vi "TouchPanel.MainTest.vi"(11 "VI ref":refnum<vi>) -> (2 "Label.Text":string, 3 "control used?":bool)   [LabVIEW 2013]
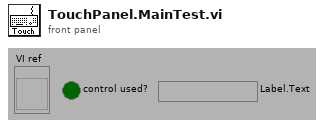
[diagram p1: front panel]
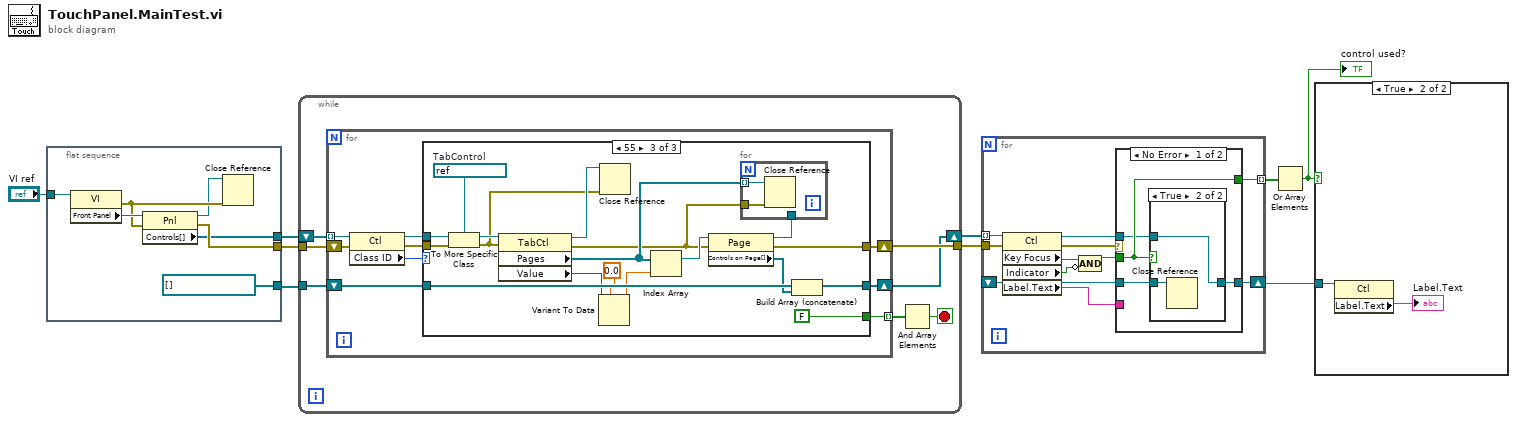
[diagram p0: block diagram]
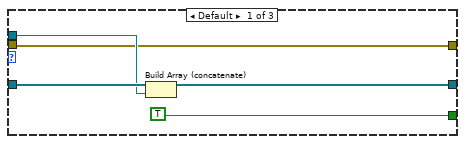
[diagram p2: hidden frame]
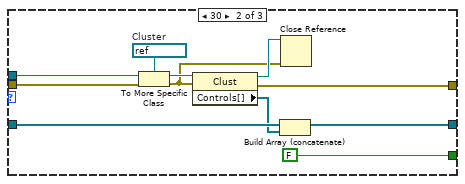
[diagram p3: hidden frame]
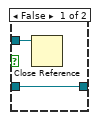
[diagram p5: hidden frame]
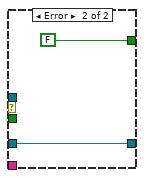
[diagram p6: hidden frame]
diagram:
  n1 = flat-sequence {
    tunnel: [w13] -> w7
    tunnel: [refnum<vi>[] []] -> w5
    tunnel: [w11] -> w4
    tunnel: "VI ref" -> [w10]
    frame #0 {
      n2 = property class="VI"(reference=w10) -> (error out=w15:errorcluster, "Front Panel"=w16:refnum<vi>)  [unwired: 1 in, 1 out]
      n3 = property class="Pnl"(reference=w16, error in=w15) -> (reference out=w14:refnum<vi>, error out=w13:errorcluster, "Controls[]"=w11:refnum<vi>[])
      n4 = Close Reference(reference=w14, error in (no error)=w15) -> ()  [unwired: 1 out]
    }
  }
  n5 = while {
    tunnel: w7 -> [w23]
    tunnel: [w22] -> w6
    tunnel: w5 -> [w21]
    shift-right: [w19] -> w3
    shift-left: w4 -> [w20]
    stop <- w17 stop-if-true
    n6 = for {
      tunnel: w20 -> [w32] mode=indexing
      shift-right: [w26] -> w22
      shift-left: w23 -> [w31]
      shift-right: [w27] -> w19
      shift-left: w21 -> [w28]
      tunnel: [w24] -> w18 mode=indexing
      n7 = property class="Ctl"(reference=w32, error in=w31) -> (reference out=w30:refnum<vi>, error out=w29:errorcluster, "Class ID"=w25:u32)
      n8 = case shown="55" w25 {
        tunnel: w30 -> [w36 w46 w65]
        tunnel: w29 -> [w34 w45 w64]
        tunnel: w28 -> [w37 w42 w60]
        tunnel: [w35 w40 w59] -> w27
        tunnel: [w34 w39 w58] -> w26
        tunnel: [TRUE FALSE FALSE] -> w24
        frame Default {
          n9 = Build Array (concatenate)(w37, w36) -> (w35:refnum<vi>[])
        }
        frame 30 {
          w47 = refnum<vi> refnum  # Cluster
          n10 = To More Specific Class(target class=w47, reference=w46, error in=w45) -> (specific class reference=w48:refnum<vi>, error out=w43:errorcluster)
          n11 = property class="Clust"(reference=w48, error in=w43) -> (reference out=w44:refnum<vi>, error out=w39:errorcluster, "Controls[]"=w41:refnum<vi>[])
          n12 = Build Array (concatenate)(w42, w41) -> (w40:refnum<vi>[])
          n13 = Close Reference(reference=w44, error in (no error)=w43) -> ()  [unwired: 1 out]
        }
        frame 55 {
          w61 = refnum<vi> refnum  # TabControl
          n14 = To More Specific Class(target class=w61, reference=w65, error in=w64) -> (specific class reference=w66:refnum<vi>, error out=w62:errorcluster)
          n15 = property class="TabCtl"(reference=w66, error in=w62) -> (reference out=w63:refnum<vi>, error out=w50:errorcluster, "Pages"=w51:refnum<vi>[], "Value"=w56:variant)
          n16 = Variant To Data(type=0.0 ("value"), Variant=w56) -> (data=w54:dbl)  [unwired: 1 in, 1 out]
          n17 = Close Reference(reference=w63, error in (no error)=w62) -> ()  [unwired: 1 out]
          n18 = Index Array(array=w51, index=w54) -> (element=w53:refnum<vi>)
          n19 = property class="Page"(reference=w53, error in=w50) -> (reference out=w49:refnum<vi>, error out=w58:errorcluster, "Controls on Page[]"=w52:refnum<vi>[])
          n20 = for {
            tunnel: w51 -> [w68] mode=indexing
            tunnel: w50 -> [w67]
            tunnel: w49 -> [_]
            n21 = Close Reference(reference=w68, error in (no error)=w67) -> ()  [unwired: 1 out]
          }
          n22 = Build Array (concatenate)(w60, w52) -> (w59:refnum<vi>[])
        }
      }
    }
    n23 = And Array Elements(Boolean array=w18) -> (logical AND=w17:bool)
  }
  n24 = for {
    tunnel: w3 -> [w79] mode=indexing
    shift-right: [w74] -> w8
    shift-left: _ -> [w76]
    tunnel: w6 -> [w78]
    tunnel: [w73] -> w9 mode=indexing
    n25 = property class="Ctl"(reference=w79, error in=w78) -> (reference out=w77:refnum<vi>, error out=w75:errorcluster, "Key Focus"=w71:bool, "Indicator"=w70:bool, "Label.Text"=w69:string)
    n26 = Compound Arithmetic op=AND(w71, invert w70) -> (w72:bool)
    n27 = case shown="No Error" w75 {
      tunnel: w77 -> [w82 _]
      tunnel: w76 -> [w81 w89]
      tunnel: w72 -> [w83 _]
      tunnel: [w80 w89] -> w74
      tunnel: [w83 FALSE ("Key Focus")] -> w73
      tunnel: w69 -> [_ _]
      frame No Error {
        n28 = case shown="True" w83 {
          tunnel: w82 -> [w85 w86]
          tunnel: w81 -> [w84 w87]
          tunnel: [w84 w86] -> w80
          frame False {
            n29 = Close Reference(reference=w85) -> ()  [unwired: 1 in, 1 out]
          }
          frame True {
            n30 = Close Reference(reference=w87) -> ()  [unwired: 1 in, 1 out]
          }
        }
      }
      frame Error {
      }
    }
  }
  n31 = Or Array Elements(Boolean array=w9) -> (logical OR=w2:bool)
  "control used?" <- w2
  n32 = case shown="True" w2 {
    tunnel: w8 -> [_ w91]
    frame False {
    }
    frame True {
      n33 = property class="Ctl"(reference=w91) -> ("Label.Text"=→"Label.Text":string)  [unwired: 1 in, 2 out]
    }
  }
